vi "Perform Bode Analysis.vi"(5 "Y Maximum (60)":dbl=60.0, 7 "Y Minimum (-60)":dbl=-60.0, 8 "error in (no error)":errorcluster, 9 "Frequency Stop (20000000: 20000000)":i32(ring)=20000000 items=["100"=100, "1000"=1000, "10000"=10000, "100000"=100000, "1000000"=1000000, "10000000"=10000000, "20000000"=20000000], 10 "Frequency Start (100: 100)":i32(ring)=100 items=["20"=20, "100"=100, "1000"=1000, "10000"=10000, "100000"=100000, "1000000"=1000000, " 10000000"=10000000], 11 "VISA resource name":refnum<visa-resource-name>) -> (0 "error out":errorcluster, 3 "VISA resource name out":refnum<visa-resource-name>)   [LabVIEW 2015, in "Agilent 2000 3000 X-Series.lvlib"]
doc: "Performs the control loop response (Bode) analysis to help you determine the margin of a control loop. \n\nA Bode plot measurement plots gain (A) in units of dB as a function of frequency. This control loop response analysis requires an input sine wave (from the oscilloscope's waveform generator, Vi) be swept from a low to a high frequency while measuring Vi and Vo RMS voltages at each step frequency, using two channels of the oscilloscope. Gain (A) at each step frequency is computed as 20Log(Vo/Vi) and plotted using a math function waveform.\n\nIt takes some time for the frequency sweep analysis to complete. You can query bit 0 of the Standard Event Status Register (*ESR?) to find out when the analysis is complete.\n\nNote:\nThis VI is not supported by EDUX1052A/G, DSOX1202A/G, DSOX1204A/G models"
uses:
  Agilent 2000 3000 X-Series.lvlib
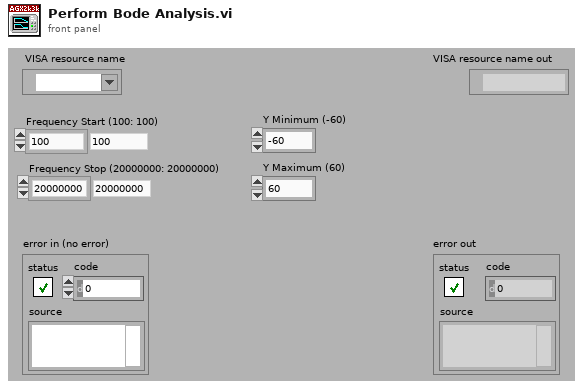
[diagram p1: front panel]
types:
  T1 = typedef "Agilent 2000 3000 X-Series.lvlib/Extended User Data.ctl" = cluster{"X-Series Mode":u16, "Acquisition Type (0: Normal)":i32}
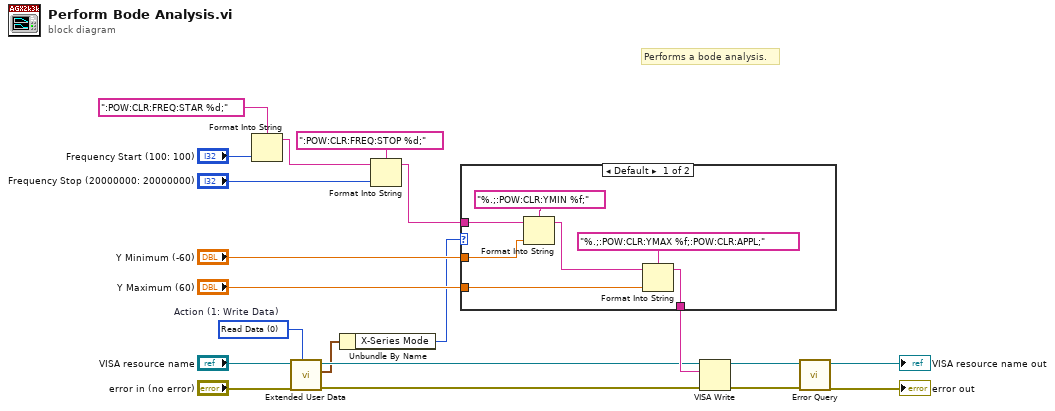
[diagram p0: block diagram]
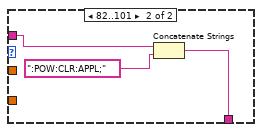
[diagram p2: hidden frame]
diagram:
  w7 = 0 items=["Read Data", "Write Data", "Clear Data", "Clear ALL Data"]  # Action (1: Write Data)
  # "Performs a bode analysis."
  n1 = Format Into String(format string=":POW:CLR:FREQ:STAR %d;", "Frequency Start (100: 100)") -> (resulting string=w12:string)  [unwired: 2 in, 1 out]
  n2 = call "Extended User Data.vi"("Action (1: Write Data)"=w7, "error in (no error)"="error in (no error)", "VISA resource name in"="VISA resource name") -> ("error out"=w3:errorcluster, "User Data Out"=w2:T1, "VISA resource name out"=w4:refnum<visa-resource-name>)  [unwired: 6 in]
  n3 = Unbundle By Name(w2) -> ("X-Series Mode"=w1:u16)
  n4 = Format Into String(format string=":POW:CLR:FREQ:STOP %d;", initial string=w12, "Frequency Stop (20000000: 20000000)") -> (resulting string=w11:string)  [unwired: 1 in, 1 out]
  n5 = case shown="Default" w1 {
    tunnel: w11 -> [w26 w30]
    tunnel: "Y Minimum (-60)" -> [w25 _]
    tunnel: "Y Maximum (60)" -> [w22 _]
    tunnel: [w21 w28] -> w8
    frame Default {
      n6 = Format Into String(format string="%.;:POW:CLR:YMIN %f;", initial string=w26, w25) -> (resulting string=w23:string)  [unwired: 1 in, 1 out]
      n7 = Format Into String(format string="%.;:POW:CLR:YMAX %f;:POW:CLR:APPL;", initial string=w23, w22) -> (resulting string=w21:string)  [unwired: 1 in, 1 out]
    }
    frame 82..101 {
      n8 = Concatenate Strings(w30, ":POW:CLR:APPL;" ("format string")) -> (w28:string)
    }
  }
  n9 = VISA Write(VISA resource name=w4, write buffer=w8, error in (no error)=w3) -> (VISA resource name out=w20:refnum<visa-resource-name>, error out=w19:errorcluster)  [unwired: 1 out]
  n10 = call "Error Query.vi"("error in (no error)"=w19, "VISA resource name"=w20) -> ("error out"=→"error out":errorcluster, "VISA resource name out"=→"VISA resource name out":refnum<visa-resource-name>)  [unwired: 8 out]
